vi "ChangeAllSeriesFileNames.vi"() -> ()   [LabVIEW 2024]
panel:
  out "error out":errorcluster
  out "current file":string
  in  "repo":path
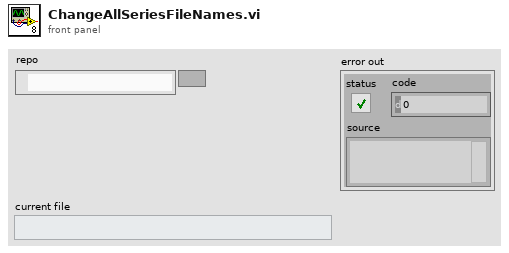
[diagram p1: front panel]
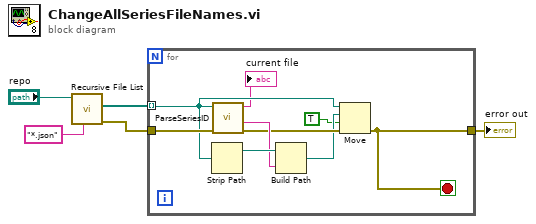
[diagram p0: block diagram]
diagram:
  n1 = call <vilib>:"Recursive File List.vi"("pattern"="*.json", "Folder Path"="repo") -> ("error out"=w2:errorcluster, "All Files in Dir"=w4:path[])  [unwired: 5 in, 3 out]
  n2 = for {
    tunnel: w4 -> [w10] mode=indexing
    tunnel: w2 -> [w14]
    tunnel: [w6] -> w1
    stop <- w6 stop-if-true
    n3 = Strip Path(path=w10) -> (stripped path=w13:path)  [unwired: 1 out]
    n4 = call "ParseSeriesID.vi"("error in"=w14, "json file path"=w10) -> ("error out"=w11:errorcluster, "filename"=w12:string, "title"=→"current file":string)  [unwired: 6 in, 1 out]
    n5 = Build Path(base path=w13, name or relative path=w12) -> (appended path=w9:path)
    n6 = Move(source path=w10, error in=w11, 9:TRUE ("overwrite (F)"), 10:w9) -> (error out=w6:errorcluster)  [unwired: 1 in, 2 out]
  }
  "error out" <- w1
